vi "Get Configuration Version.vi"(8 "error in (no error)":errorcluster, 11 "Item Ref in":T2 format="%.0x") -> (0 "error out":errorcluster, 2 "version":T1, 3 "Item Ref out":T2 format="%.0x")   [LabVIEW 2019, in "DSF Shared.lvlib"]
uses:
  DSF Shared.lvlib
  <vilib>/NI VeriStand/Custom Device API/Custom Device API.lvlib
  DSF Core.lvlibp/Typedefs/DSF Version Info.ctl
  <vilib>/NI VeriStand/Custom Device API/Get Item Property (Variant).vi
  <vilib>/NI VeriStand/Custom Device API/Custom Device Item Ref.ctl
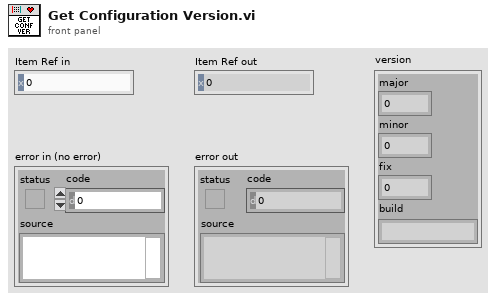
[diagram p1: front panel]
types:
  T1 = typedef "DSF Core.lvlibp/DSF Version Info.ctl" = cluster{"major":u32, "minor":u32, "fix":u32, "build":string}
  T2 = typedef "Custom Device API.lvlib/Custom Device Item Ref.ctl" = u64
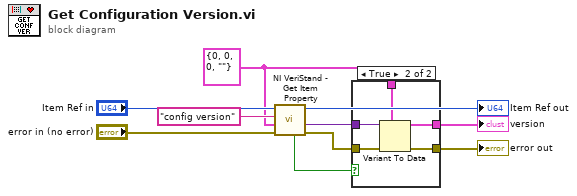
[diagram p0: block diagram]
diagram:
  w2 = T1 {"major"=0, "minor"=0, "fix"=0, "build"=""} ("version")
  n1 = call-poly <vilib>:"NI VeriStand - Get Item Property.vi"("error in (no error)"="error in (no error)", "Default Value"=w2, "Property Name"="config version" ("dsf options"), "Item Ref in"="Item Ref in") -> ("error out"=w8:errorcluster, "Value"=w7:variant, "Item Ref out"=→"Item Ref out":T2, "Found?"=w4:bool)  [unwired: 4 in]
  n2 = case shown="True" w4 {
    tunnel: w8 -> [w11 w17]
    tunnel: w2 -> [w12 w16]
    tunnel: w7 -> [_ w15]
    tunnel: [w11 w14] -> w6
    tunnel: [w12 w13] -> w1
    frame False {
    }
    frame True {
      n3 = Variant To Data(error in=w17, type=w16, Variant=w15) -> (data=w13:T1, error out=w14:errorcluster)
    }
  }
  "error out" <- w6
  "version" <- w1
